vi "Equal - CM,CM.vi"(1 "Complex Matrix B":T1, 2 "Complex Matrix A":T1) -> (0 "A = B?":bool)   [LabVIEW 2017, in "NI_Matrix.lvlib"]
doc: "Returns TRUE if <B>x</B> is equal to <B>y</B>. Otherwise, this function returns FALSE."
uses:
  <vilib>/Analysis/Matrix/NI_Matrix.lvlib
  <vilib>/Analysis/Matrix/Datatypes/ComplexMatrix.ctl
  <vilib>/Analysis/Matrix/Numeric/Conversions/Matrix To Array - CM.vi
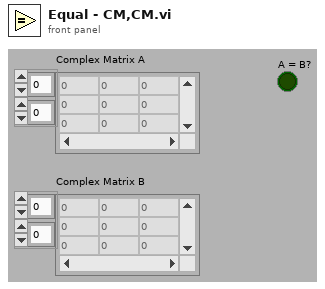
[diagram p1: front panel]
types:
  T1 = typedef "NI_Matrix.lvlib/ComplexMatrix.ctl" = cdb[][]
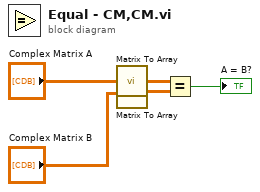
[diagram p0: block diagram]
diagram:
  n1 = call-poly <vilib>:"Matrix To Array.vi"("Complex Matrix"="Complex Matrix A") -> ("Complex 2D Array"=w3:cdb[][])
  n2 = call-poly <vilib>:"Matrix To Array.vi"("Complex Matrix"="Complex Matrix B") -> ("Complex 2D Array"=w2:cdb[][])
  n3 = Equal?(x=w3, y=w2) -> (x = y?=→"A = B?":bool)
